vi "PH_gentec_M-Link.Action set Settings.vi"(0 "i ref in":refnum<vi>, 5 "error in":errorcluster) -> (14 "i ref out":refnum<vi>, 19 "error out":errorcluster)   [LabVIEW 2014, in "PH_gentec_M-Link.lvlib"]
doc: "This VI sets the device to the wanted settings."
uses:
  PH_gentec_M-Link.lvlib
  PH_Basics/PH_Powermeter_BaseClass/PH_Powermeter_BaseClass.State.ctl
  PH_Basics/PH_Powermeter_BaseClass/PH_Powermeter_BaseClass.lvlib
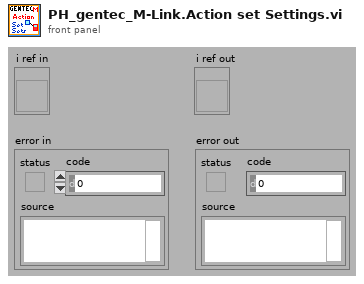
[diagram p1: front panel]
types:
  T1 = typedef "PH_Powermeter_BaseClass.lvlib/PH_Powermeter_BaseClass.State.ctl" = enum32{"off", "operating", "opened", "checked", "connected", "Sets to change", "running"}
  T2 = typedef "PH_Powermeter_BaseClass.lvlib/PH_Powermeter_BaseClass.i attribute.ctl" = cluster{"GUI References":T3, "Connection":T4, "Head Attributes":T5, "VISA resource":refnum<visa-resource-name>, "Energy":T6, "Service ID Energy":i32, "Wanted Settings":T7, "Current Settings":T7}
  T3 = typedef "PH_Powermeter_BaseClass.lvlib/PH_Powermeter_BaseClass.GUI Refs.ctl" = cluster{"Head Attributes":refnum<vi>, "Energy":refnum<vi>, "Connection":refnum<vi>, "VISA Resource":refnum<vi>, "Scaling Factor":refnum<vi>, "Range":refnum<vi>, "Wavelength":refnum<vi>, "Trigger Level":refnum<vi>, "Wanted Settings":refnum<vi>, "Current Settings":refnum<vi>}
  T4 = typedef "PH_Powermeter_BaseClass.lvlib/PH_Powermeter_BaseClass.Connection.ctl" = cluster{"failed checks":i8, "Timeout":bool, "Data read":string, "Failure":bool, "Error":bool, "State":T1}
  T5 = typedef "PH_Powermeter_BaseClass.lvlib/PH_Powermeter_BaseClass.Head Attributes.ctl" = cluster{"Instrument Type":string, "Head Version":string, "Head Name":string, "Serial Number":string, "Firmware":string, "Sensor Type":string, "MinimumRange":u32, "Maximum Range":u32, "Min Wavelength":i32, "Max Wavelength":i32}
  T6 = typedef "PH_Powermeter_BaseClass.lvlib/PH_Powermeter_BaseClass.Energy.ctl" = cluster{"current Value":dbl, "unscaled":dbl, "Scaling Factor":dbl}
  T7 = typedef "PH_Powermeter_BaseClass.lvlib/PH_gentec_BaseClass.Head Settings.ctl" = cluster{"Trigger Level":dbl, "Wavelength":u32, "Range":u32}
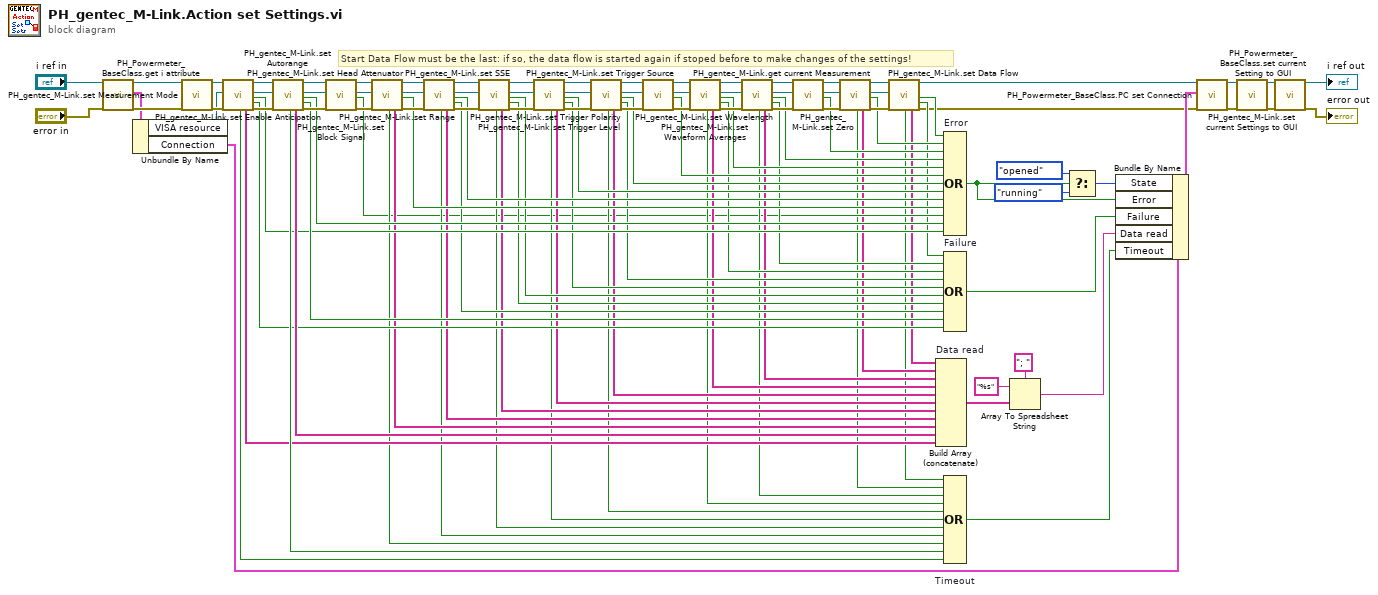
[diagram p0: block diagram]
diagram:
  # "Start Data Flow must be the last: if so, the data flow is started again if stoped before to make changes of the settings!"
  n1 = call "PH_Powermeter_BaseClass.get i attribute.vi"("i ref in"="i ref in", "error in (no error)"="error in") -> ("i ref out"=w12:refnum<vi>, "i attribute"=w9:T2, "error out"=w10:errorcluster)  [unwired: 15 in]
  n2 = Unbundle By Name(w9) -> ("VISA resource"=w8:refnum<visa-resource-name>, "Connection"=w7:T4)
  n3 = call "PH_gentec_M-Link.set Measurement Mode.vi"("i ref in"=w12, "error in"=w10) -> ("i ref out"=w109:refnum<vi>, "error out"=w111:errorcluster)  [unwired: 16 in]
  n4 = call "PH_gentec_M-Link.set Enable Anticipation.vi"("i ref in"=w109, "VISA resource in"=w8, "error in"=w111) -> ("Timeout"=w94:bool, "Data read"=w95:string[], "i ref out"=w108:refnum<vi>, "VISA resource out"=w107:refnum<visa-resource-name>, "Error"=w92:bool, "Failure"=w93:bool, "error out"=w110:errorcluster)  [unwired: 10 in]
  n5 = call "PH_gentec_M-Link.set Autorange.vi"("i ref in"=w108, "VISA resource in"=w107, "error in"=w110) -> ("Timeout"=w105:bool, "Data read"=w100:string[], "i ref out"=w97:refnum<vi>, "VISA resource out"=w96:refnum<visa-resource-name>, "Error"=w103:bool, "Failure"=w102:bool, "error out"=w106:errorcluster)  [unwired: 10 in]
  n6 = call "PH_gentec_M-Link.set Block Signal.vi"("i ref in"=w97, "VISA resource in"=w96, "error in"=w106) -> ("i ref out"=w90:refnum<vi>, "VISA resource out"=w89:refnum<visa-resource-name>, "Error"=w33:bool, "error out"=w98:errorcluster)  [unwired: 13 in]
  n7 = call "PH_gentec_M-Link.set Head Attenuator.vi"("i ref in"=w90, "VISA resource in"=w89, "error in"=w98) -> ("Timeout"=w88:bool, "Data read"=w87:string[], "i ref out"=w23:refnum<vi>, "VISA resource out"=w84:refnum<visa-resource-name>, "Error"=w86:bool, "error out"=w91:errorcluster)  [unwired: 11 in]
  n8 = call "PH_gentec_M-Link.set Range.vi"("i ref in"=w23, "VISA resource in"=w84, "error in"=w91) -> ("Timeout"=w83:bool, "Data read"=w82:string[], "i ref out"=w78:refnum<vi>, "VISA resource out"=w77:refnum<visa-resource-name>, "Error"=w80:bool, "Failure"=w81:bool, "error out"=w85:errorcluster)  [unwired: 10 in]
  n9 = call "PH_gentec_M-Link.set SSE.vi"("i ref in"=w78, "VISA resource in"=w77, "error in"=w85) -> ("Timeout"=w76:bool, "Data read"=w75:string[], "i ref out"=w71:refnum<vi>, "VISA resource out"=w70:refnum<visa-resource-name>, "Error"=w73:bool, "Failure"=w74:bool, "error out"=w79:errorcluster)  [unwired: 10 in]
  n10 = call "PH_gentec_M-Link.set Trigger Level.vi"("i ref in"=w71, "VISA resource in"=w70, "error in"=w79) -> ("Timeout"=w66:bool, "Data read"=w67:string[], "i ref out"=w64:refnum<vi>, "VISA resource out"=w63:refnum<visa-resource-name>, "Error"=w69:bool, "Failure"=w68:bool, "error out"=w72:errorcluster)  [unwired: 10 in]
  n11 = call "PH_gentec_M-Link.set Trigger Polarity.vi"("i ref in"=w64, "VISA resource in"=w63, "error in"=w72) -> ("Timeout"=w59:bool, "Data read"=w60:string[], "i ref out"=w57:refnum<vi>, "VISA resource out"=w56:refnum<visa-resource-name>, "Error"=w62:bool, "Failure"=w61:bool, "error out"=w65:errorcluster)  [unwired: 10 in]
  n12 = call "PH_gentec_M-Link.set Trigger Source.vi"("i ref in"=w57, "VISA resource in"=w56, "error in"=w65) -> ("i ref out"=w53:refnum<vi>, "VISA resource out"=w52:refnum<visa-resource-name>, "Error"=w55:bool, "error out"=w58:errorcluster)  [unwired: 13 in]
  n13 = call "PH_gentec_M-Link.set Waveform Averages.vi"("i ref in"=w53, "VISA resource in"=w52, "error in"=w58) -> ("Timeout"=w51:bool, "Data read"=w50:string[], "i ref out"=w46:refnum<vi>, "VISA resource out"=w45:refnum<visa-resource-name>, "Error"=w48:bool, "Failure"=w49:bool, "error out"=w54:errorcluster)  [unwired: 10 in]
  n14 = call "PH_gentec_M-Link.set Wavelength.vi"("i ref in"=w46, "VISA resource in"=w45, "error in"=w54) -> ("Timeout"=w44:bool, "Data read"=w43:string[], "i ref out"=w38:refnum<vi>, "VISA resource out"=w39:refnum<visa-resource-name>, "Error"=w41:bool, "Failure"=w42:bool, "error out"=w47:errorcluster)  [unwired: 10 in]
  n15 = call "PH_gentec_M-Link.set Zero.vi"("i ref in"=w38, "VISA resource in"=w39, "error in"=w47) -> ("i ref out"=w35:refnum<vi>, "VISA resource out"=w34:refnum<visa-resource-name>, "Error"=w37:bool, "error out"=w40:errorcluster)  [unwired: 13 in]
  n16 = call "PH_gentec_M-Link.get current Measurement.vi"("i ref in"=w35, "VISA resource in"=w34, "error in"=w40) -> ("Timeout"=w32:bool, "Data read"=w31:string[], "i ref out"=w29:refnum<vi>, "VISA resource out"=w28:refnum<visa-resource-name>, "Error"=w30:bool, "error out"=w36:errorcluster)  [unwired: 11 in]
  n17 = call "PH_gentec_M-Link.set Data Flow.vi"("i ref in"=w29, "VISA resource in"=w28, "error in"=w36) -> ("Timeout"=w27:bool, "Data read"=w24:string[], "i ref out"=w18:refnum<vi>, "Error"=w26:bool, "Failure"=w25:bool, "error out"=w17:errorcluster)  [unwired: 10 in, 1 out]
  n18 = Build Array (concatenate) "Data read"(w24, w31, w43, w50, w60, w67, w75, w82, w87, w100, w95) -> (w99:string[])
  n19 = Compound Arithmetic op=OR "Error"(w26, w30, w37, w41, w48, w55, w62, w69, w80, w86, w33, w103, w92) -> (w16:bool)
  n20 = Compound Arithmetic op=OR "Failure"(w25, w42, w49, w61, w68, w73, w74, w81, w102, w93) -> (w101:bool)
  n21 = Compound Arithmetic op=OR "Timeout"(w27, w32, w44, w51, w59, w66, w76, w83, w88, w105, w94) -> (w104:bool)
  n22 = Array To Spreadsheet String(delimiter (Tab)="; ", array=w99, 3:"%s" ("format string")) -> (spreadsheet string=w20:string)
  n23 = Select(t=PH_Powermeter_BaseClass.State."opened" ("State"), s=w16, f=PH_Powermeter_BaseClass.State."running") -> (s? t:f=w14:T1)
  n24 = Bundle By Name(cluster=w7, "State"=w14, "Error"=w16, "Failure"=w101, "Data read"=w20, "Timeout"=w104) -> (w19:T4)
  n25 = call "PH_Powermeter_BaseClass.PC set Connection.vi"("VI in"=w18, "Connection"=w19, "error in (no error)"=w17) -> ("VI out"=w6:refnum<vi>, "error out"=w4:errorcluster)  [unwired: 15 in]
  n26 = call "PH_gentec_M-Link.set current Settings to GUI.vi"("i ref in"=w6, "error in"=w4) -> ("i ref out"=w2:refnum<vi>, "error out"=w5:errorcluster)  [unwired: 16 in]
  n27 = call "PH_Powermeter_BaseClass.set current Setting to GUI.vi"("VI in"=w2, "error in (no error)"=w5) -> ("VI out"=→"i ref out":refnum<vi>, "error out"=→"error out":errorcluster)  [unwired: 16 in]
